vi "Temp Graph Update.vi"(5 "Property Name":T8, 6 "State":T10=enum."Update Graph", 7 "Data Name":T9, 8 "error in (no error)":errorcluster, 11 "Property In":variant) -> (0 "error out":errorcluster, 3 "Item Strings":string[](array[string]))   [LabVIEW 2020, in "2D Plot.lvclass"]
uses:
  <vilib>/Math Plots/2D Math Plots/2D Plot/2D Plot/2D Plot.lvclass
  <vilib>/Math Plots/2D Math Plots/2D Plot/2D Plot/Typedef/Temp Graph State.ctl
  <vilib>/Math Plots/2D Math Plots/2D Plot/2D Plot/Typedef/Temp Graph Data Action.ctl
  <vilib>/Math Plots/2D Math Plots/2D Plot/2D Plot/Typedef/Temp Graph Property Action.ctl
  <vilib>/Math Plots/2D Math Plots/2D Plot/2D Plot/Typedef/Multiplot Representation.ctl
  <vilib>/Math Plots/2D Math Plots/2D Plot/2D Plot/Typedef/Plot Representation.ctl
  <vilib>/Math Plots/2D Math Plots/2D Plot/2D Plot/Typedef/Range Cluster.ctl
  <vilib>/Math Plots/2D Math Plots/2D Plot/2D Plot/Typedef/Scale Array.ctl
  <vilib>/Math Plots/2D Math Plots/2D Plot/2D Plot/Typedef/Scale Cluster.ctl
  <vilib>/Utility/miscctls.llb/LVOffsetAndMultiplierTypeDef.ctl
  <vilib>/Math Plots/2D Math Plots/2D Plot/2D Plot/Typedef/Graph General Property.ctl
  <vilib>/Math Plots/2D Math Plots/2D Plot/Action String/2DMathPlot Ctrl Act Queue.ctl
  <vilib>/Math Plots/2D Math Plots/2D Plot/Action String/2DMathPlot Ctrl Act Cluster.ctl
  <vilib>/Math Plots/2D Math Plots/2D Plot/Action String/2DMathPlot State Class.ctl
  <vilib>/Math Plots/2D Math Plots/2D Plot/2D Plot/2D Plot.lvclass/2D Plot.ctl
panel:
  in  "Graph General":T1
  in  "Format Property":string[](array[string])
  in  "Scale Array":T2
  in  "Multiplot Representation":T5
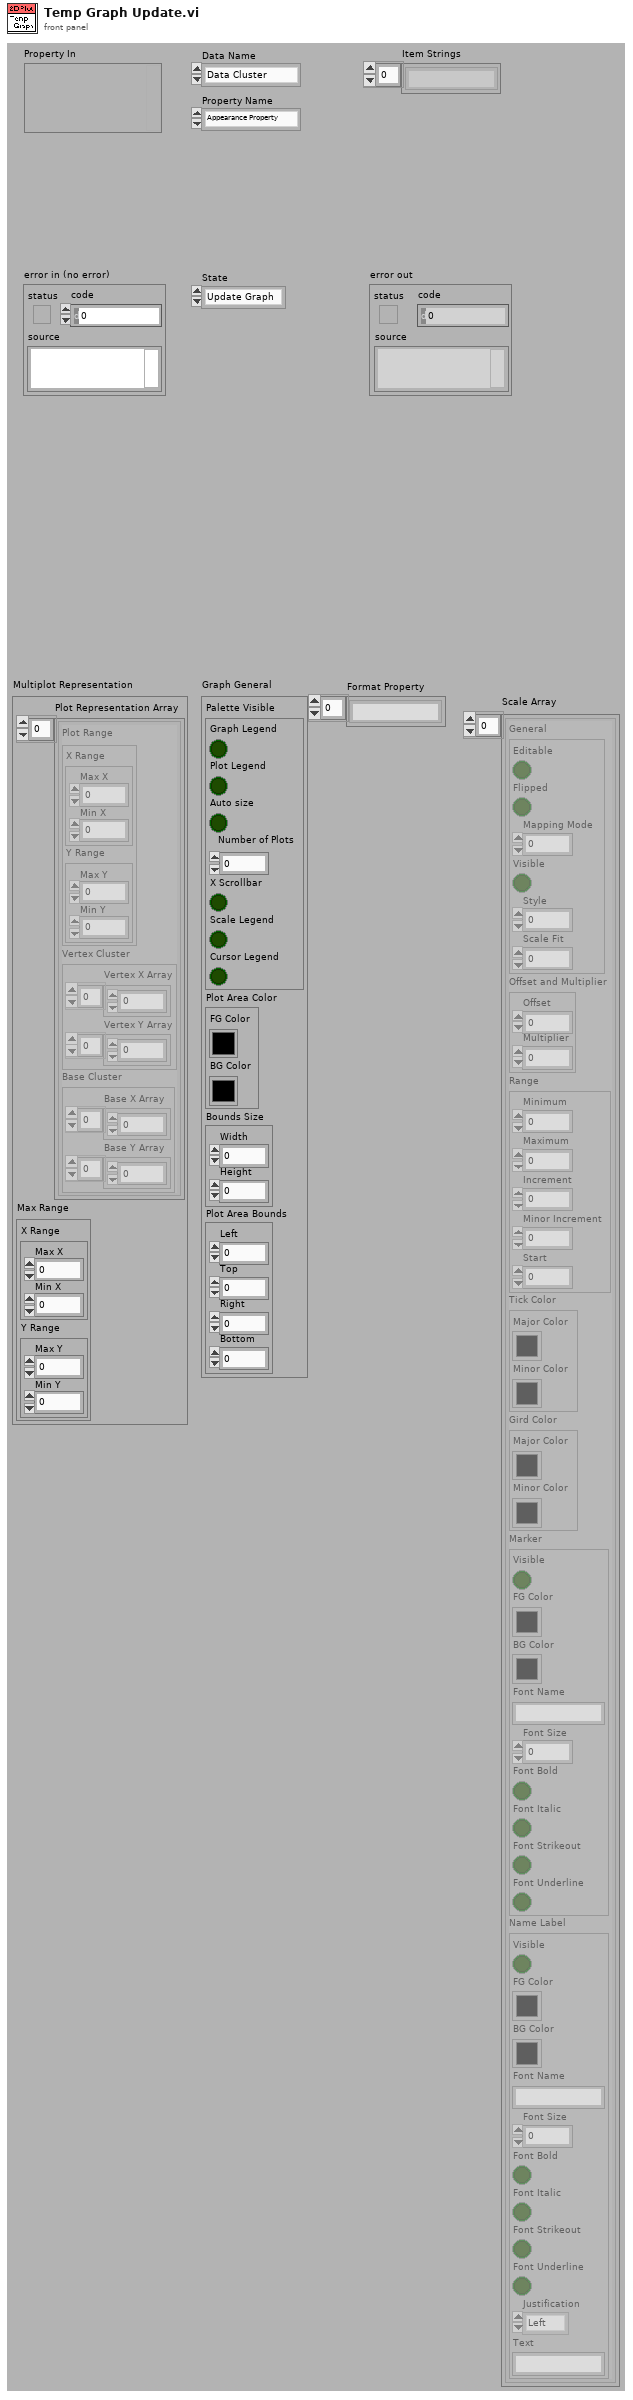
[diagram p1: front panel]
types:
  T1 = typedef "2D Plot.lvclass/Graph General Property.ctl" = cluster{"Palette Visible":cluster{"Graph Legend":bool, "Plot Legend":bool, "Auto size":bool, "Number of Plots":u32, "X Scrollbar":bool, "Scale Legend":bool, "Cursor Legend":bool}, "Plot Area Color":cluster{"FG Color":u32, "BG Color":u32}, "Bounds Size":cluster{"Width":u32, "Height":u32}, "Plot Area Bounds":cluster{"Left":i16, "Top":i16, "Right":i16, "Bottom":i16}}
  T2 = typedef "2D Plot.lvclass/Scale Array.ctl" = T3[]
  T3 = typedef "2D Plot.lvclass/Scale Cluster.ctl" = cluster{"General":cluster{"Editable":bool, "Flipped":bool, "Mapping Mode":u8, "Visible":bool, "Style":u8, "Scale Fit":u8}, "Offset and Multiplier":T4, "Range":cluster{"Minimum":dbl, "Maximum":dbl, "Increment":dbl, "Minor Increment":dbl, "Start":dbl}, "Tick Color":cluster{"Major Color":u32, "Minor Color":u32}, "Gird Color":cluster{"Major Color":u32, "Minor Color":u32}, "Marker":cluster{"Visible":bool, "FG Color":u32, "BG Color":u32, "Font Name":string, "Font Size":u32, "Font Bold":bool, "Font Italic":bool, "Font Strikeout":bool, "Font Underline":bool}, "Name Label":cluster{"Visible":bool, "FG Color":u32, "BG Color":u32, "Font Name":string, "Font Size":u32, "Font Bold":bool, "Font Italic":bool, "Font Strikeout":bool, "Font Underline":bool, "Justification":enum16{"Left", "Center", "Right"}, "Text":string}}
  T4 = typedef "LVOffsetAndMultiplierTypeDef.ctl" = cluster{"Offset":dbl, "Multiplier":dbl}
  T5 = typedef "2D Plot.lvclass/Multiplot Representation.ctl" = cluster{"Plot Representation Array":T6[], "Max Range":T7}
  T6 = typedef "2D Plot.lvclass/Plot Representation.ctl" = cluster{"Plot Range":T7, "Vertex Cluster":cluster{"Vertex X Array":dbl[], "Vertex Y Array":dbl[]}, "Base Cluster":cluster{"Base X Array":dbl[], "Base Y Array":dbl[]}}
  T7 = typedef "2D Plot.lvclass/Range Cluster.ctl" = cluster{"X Range":cluster{"Max X":dbl, "Min X":dbl}, "Y Range":cluster{"Max Y":dbl, "Min Y":dbl}}
  T8 = typedef "2D Plot.lvclass/Temp Graph Property Action.ctl" = enum16{"Appearance Property", "Format Property", "Plots Property", "Scales Property"}
  T9 = typedef "2D Plot.lvclass/Temp Graph Data Action.ctl" = enum16{"Data Cluster", "Property Class", "Control Queue"}
  T10 = typedef "2D Plot.lvclass/Temp Graph State.ctl" = enum16{"Create", "Update Graph", "Update Property Only", "Get Plot Name", "Get Axis Name", "Destory"}
  T11 = typedef "2DMathPlot Ctrl Act Queue.ctl" = refnum<queue>
  T12 = typedef "2DMathPlot State Class.ctl" = enum16{"Update All (Undo)", "Update General", "Update Appearance", "Update Format", "Update Scale", "Update Marker", "Update Cursor", "None"}
  T13 = typedef "2D Plot.lvclass/Plot Property Array.ctl" = T14[]
  T14 = typedef "2D Plot.lvclass/Plot Property.ctl" = cluster{"Bar Plot Style":u8, "DigitalLineStyle":u8, "TransitionLocation":u8, "Transition Type":u8, "Fill To":i16, "Fill/Pt. Color":u32, "Label Style":u8, "Line Style":u8, "Line Width":u8, "Plot Color":u32, "Plot Interpolation":u8, "Plot Name":string, "Point Style":u8, "Visible?":bool, "XScaleIdx":u32, "YScaleIdx":u32}
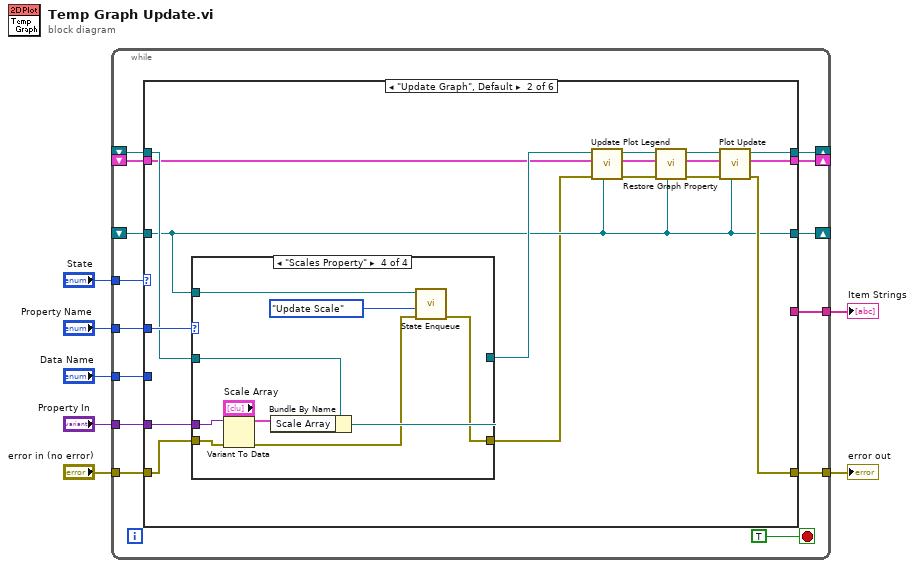
[diagram p0: block diagram]
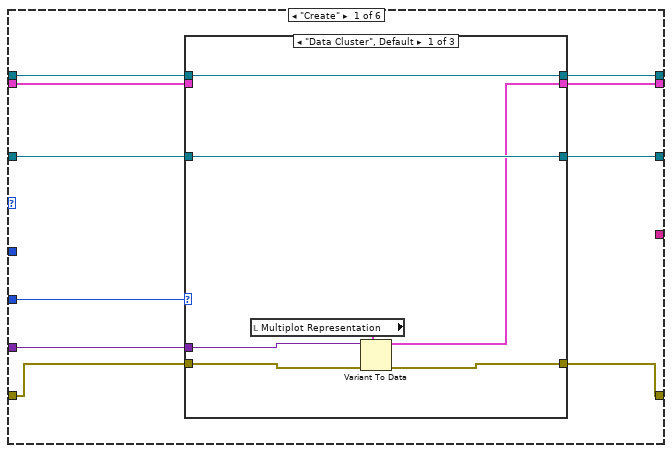
[diagram p2: hidden frame]
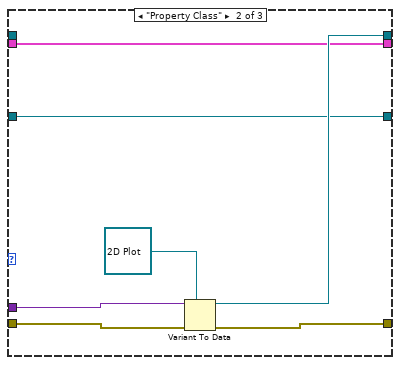
[diagram p3: hidden frame]
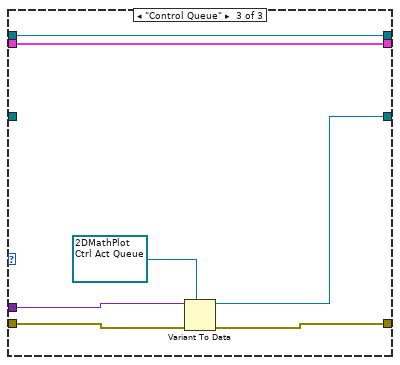
[diagram p4: hidden frame]
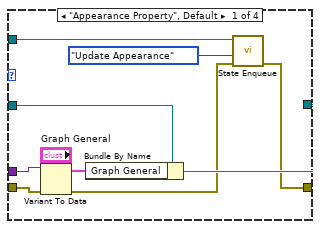
[diagram p5: hidden frame]
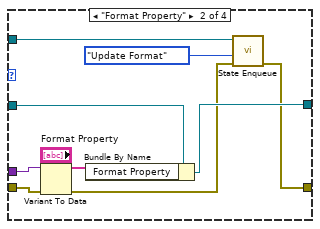
[diagram p6: hidden frame]
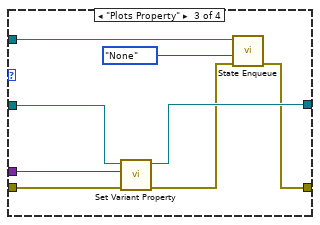
[diagram p7: hidden frame]
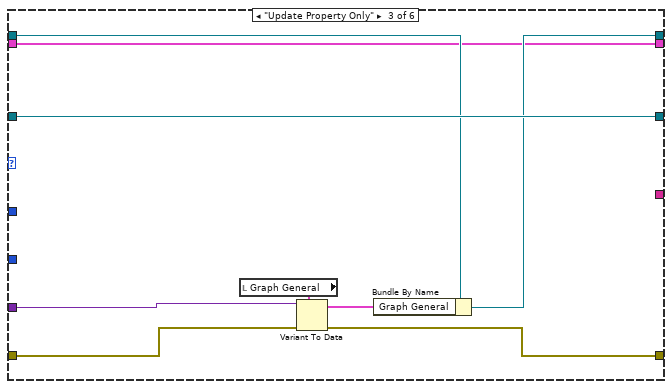
[diagram p8: hidden frame]
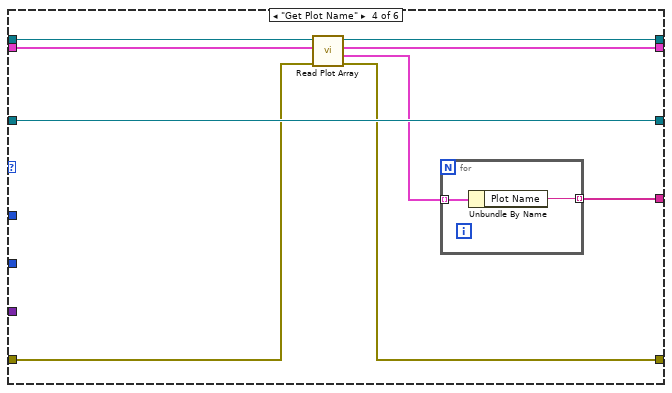
[diagram p9: hidden frame]
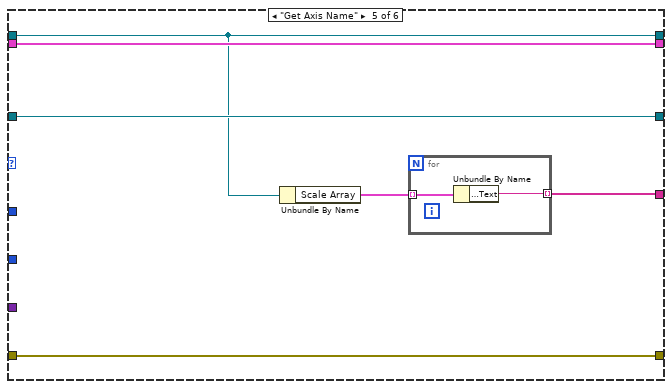
[diagram p10: hidden frame]
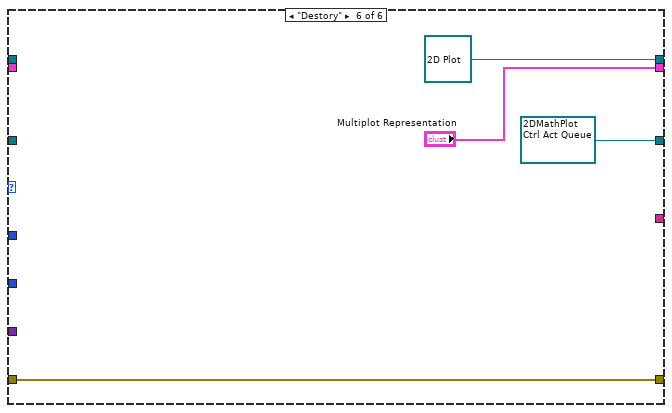
[diagram p11: hidden frame]
diagram:
  n1 = while {
    tunnel: "State" -> [w21]
    tunnel: "Property In" -> [w20]
    tunnel: "Property Name" -> [w19]
    tunnel: "Data Name" -> [w18]
    tunnel: "error in (no error)" -> [w17]
    tunnel: [w16] -> w2
    shift-right: [w14] -> _
    shift-left: _ -> [w13]
    shift-right: [w15] -> _
    shift-left: _ -> [w12]
    shift-right: [w11] -> _
    shift-left: _ -> [w10]
    tunnel: [w8] -> w1
    stop <- TRUE stop-if-true
    n2 = case shown="\"Update Graph\", Default" w21 {
      tunnel: w20 -> [w30 w68 w107 _ _ _]
      tunnel: w19 -> [_ w67 _ _ _ _]
      tunnel: w18 -> [w31 _ _ _ _ _]
      tunnel: w17 -> [w29 w66 w114 w119 w129 w134]
      tunnel: [w24 w60 w113 w118 w129 w134] -> w16
      tunnel: [w26 w62 w109 w120 w128 refnum<class "2D Plot.lvclass"> refnum ("2D Plot.lvclass")] -> w15
      tunnel: [w25 w55 w112 w122 w130 T11 refnum ("Control Ref Queue")] -> w14
      tunnel: w13 -> [w27 w55 w112 w122 w130 _]
      tunnel: w12 -> [w28 w65 w110 w121 w128 _]
      tunnel: [w23 w63 w108 w123 w131 "Multiplot Representation"] -> w11
      tunnel: w10 -> [w22 w57 w108 w123 w131 _]
      tunnel: [_ _ _ w116 w126 _] -> w8
      frame "Create" {
        n3 = case shown="\"Data Cluster\", Default" w31 {
          tunnel: w30 -> [w38 w45 w52]
          tunnel: w29 -> [w37 w44 w51]
          tunnel: w28 -> [w35 _ w48]
          tunnel: w27 -> [w36 w42 _]
          tunnel: [w35 w43 w48] -> w26
          tunnel: [w36 w42 w49] -> w25
          tunnel: [w34 w40 w47] -> w24
          tunnel: [w33 w39 w46] -> w23
          tunnel: w22 -> [_ w39 w46]
          frame "Data Cluster", Default {
            n4 = local read "Multiplot Representation"() -> (w32:T5)
            n5 = Variant To Data(error in=w37, type=w32, Variant=w38) -> (data=w33:T5, error out=w34:errorcluster)
          }
          frame "Property Class" {
            n6 = Variant To Data(error in=w44, type=refnum<class "2D Plot.lvclass"> refnum ("2D Plot.lvclass"), Variant=w45) -> (data=w43:refnum<class "2D Plot.lvclass">, error out=w40:errorcluster)
          }
          frame "Control Queue" {
            n7 = Variant To Data(error in=w51, type=T11 refnum ("Control Ref Queue"), Variant=w52) -> (data=w49:T11, error out=w47:errorcluster)
          }
        }
      }
      frame "Update Graph", Default {
        n8 = case shown="\"Scales Property\"" w67 {
          tunnel: w68 -> [w76 w88 w93 w106]
          tunnel: w66 -> [w77 w87 w94 w105]
          tunnel: [w69 w80 w89 w97] -> w53
          tunnel: w65 -> [w78 w84 w96 w104]
          tunnel: [w75 w83 w95 w103] -> w58
          tunnel: w55 -> [w71 w82 w91 w99]
          frame "Appearance Property", Default {
            n9 = Variant To Data(error in=w77, type="Graph General", Variant=w76) -> (data=w73:T1, error out=w70:errorcluster)
            n10 = Bundle By Name(cluster=w78, "Graph General"=w73) -> (w75:refnum<class "2D Plot.lvclass">)
            n11 = call <vilib>:"State Enqueue.vi"("error in (no error)"=w70, "Display State Change Class"=2DMathPlot_State_Class."Update Appearance", "Control Ref Queue"=w71) -> ("error out"=w69:errorcluster)  [unwired: 8 out]
          }
          frame "Format Property" {
            n12 = Variant To Data(error in=w87, type="Format Property", Variant=w88) -> (data=w86:string[], error out=w81:errorcluster)
            n13 = Bundle By Name(cluster=w84, "Format Property"=w86) -> (w83:refnum<class "2D Plot.lvclass">)
            n14 = call <vilib>:"State Enqueue.vi"("error in (no error)"=w81, "Display State Change Class"=2DMathPlot_State_Class."Update Format", "Control Ref Queue"=w82) -> ("error out"=w80:errorcluster)  [unwired: 8 out]
          }
          frame "Plots Property" {
            n15 = call-dynamic "Set Variant Property.vi"("error in (no error)"=w94, "Property In"=w93, "2D Plot.lvclass"=w96) -> ("error out"=w90:errorcluster, "2D Plot.lvclass"=w95:refnum<class "2D Plot.lvclass">)  [unwired: 1 in, 6 out]
            n16 = call <vilib>:"State Enqueue.vi"("error in (no error)"=w90, "Display State Change Class"=2DMathPlot_State_Class."None", "Control Ref Queue"=w91) -> ("error out"=w89:errorcluster)  [unwired: 8 out]
          }
          frame "Scales Property" {
            n17 = Variant To Data(error in=w105, type="Scale Array", Variant=w106) -> (data=w101:T2, error out=w98:errorcluster)
            n18 = Bundle By Name(cluster=w104, "Scale Array"=w101) -> (w103:refnum<class "2D Plot.lvclass">)
            n19 = call <vilib>:"State Enqueue.vi"("error in (no error)"=w98, "Display State Change Class"=2DMathPlot_State_Class."Update Scale", "Control Ref Queue"=w99) -> ("error out"=w97:errorcluster)  [unwired: 8 out]
          }
        }
        n20 = call <vilib>:"Update Plot Legend.vi"("Control Ref Queue"=w55, "error in (no error)"=w53, "Multiplot Representation In"=w57, "2D Plot in"=w58) -> ("error out"=w54:errorcluster, "Multiplot Representation Out"=w56:T5, "2D Plot out"=w59:refnum<class "2D Plot.lvclass">)  [unwired: 5 out]
        n21 = call-dynamic "Restore Graph Property.vi"("Control Ref Queue"=w55, "error in (no error)"=w54, "2D Plot.lvclass in"=w59) -> ("error out"=w61:errorcluster, "2D Plot.lvclass out"=w64:refnum<class "2D Plot.lvclass">)  [unwired: 1 in, 6 out]
        n22 = call <vilib>:"Plot Update.vi"("Control Ref Queue"=w55, "error in (no error)"=w61, "Multiplot Representation In"=w56, "2D Plot.lvclass in"=w64) -> ("error out"=w60:errorcluster, "Multiplot Representation Out"=w63:T5, "2D Plot.lvclass out"=w62:refnum<class "2D Plot.lvclass">)  [unwired: 5 out]
      }
      frame "Update Property Only" {
        n23 = local read "Graph General"() -> (w111:T1)
        n24 = Variant To Data(error in=w114, type=w111, Variant=w107) -> (data=w115:T1, error out=w113:errorcluster)
        n25 = Bundle By Name(cluster=w110, "Graph General"=w115) -> (w109:refnum<class "2D Plot.lvclass">)
      }
      frame "Get Plot Name" {
        n26 = call-dynamic "Read Plot Array.vi"("error in (no error)"=w119, "2D Plot in"=w121) -> ("error out"=w118:errorcluster, "Plot Property Array"=w117:T13, "2D Plot out"=w120:refnum<class "2D Plot.lvclass">)  [unwired: 7 out]
        n27 = for {
          tunnel: w117 -> [w125] mode=indexing
          tunnel: [w124] -> w116 mode=indexing
          n28 = Unbundle By Name(w125) -> ("Plot Name"=w124:string)
        }
      }
      frame "Get Axis Name" {
        n29 = Unbundle By Name(w128) -> ("Scale Array"=w127:T2)
        n30 = for {
          tunnel: w127 -> [w133] mode=indexing
          tunnel: [w132] -> w126 mode=indexing
          n31 = Unbundle By Name(w133) -> ("Name Label.Text"=w132:string)
        }
      }
      frame "Destory" {
      }
    }
  }
  "error out" <- w2
  "Item Strings" <- w1
